vi "PMOD Example(FPGA).vi"() -> ()   [LabVIEW 2014]
uses:
  Controls/SPIExample.CurrentStateFPGA.ctl
  <userlib>/_NI SPI IP/FPGA/Controllers/Public/Transfer Settings.ctl
  vi.lib/SPIAPI/Controls/SPI Settings.ctl
  vi.lib/SPIAPI/Controls/Signal Properties.ctl
  <vilib>/rvi/Emulation/niFpgaGetClockAttributes.vi
  <vilib>/rvi/Emulation/niFpgaSctlEmulationGetInTimedLoop.vi
  <vilib>/rvi/Emulation/niFpgaEmulationReportErrorSimple.vi
  <vilib>/rvi/Emulation/niFpgaProcessEmulError.vi
  <vilib>/rvi/interface/RandomDataEmulation/niFpgaRandomDataHandleErrors.vi
  <vilib>/rvi/Emulation/niFpgaCriticalErrorInLSC.vi
  <vilib>/rvi/DataTransferAndStorage/Container/XNode/niFpgaContainer.xnode
  <vilib>/rvi/interface/RandomDataEmulation/nirviRandomDataFpgaReadWriteTemplate.vi
  <userlib>/_NI SPI IP/FPGA/Controllers/NI SPI IP FPGA.lvlib
panel:
  out "Raw ADC Data":u64
  out "read Iterations":i32
  in  "Data To ADC":u64=2147483648
  in  "Chip Select":u8
  in  "SPI PHY Settings":T1={"Divide Value"=20, "Transfer Length (bits)"=32, "CS Asserted Polarity"=FALSE, "Clock Polarity (CPOL)"=FALSE, "Clock Phase (CPHA)"=FALSE, "Lengthen MISO Setup"=FALSE, "Direction Change Bit"=0, "MOSI Starts as Output"=FALSE, "Tristatable MOSI"=FALSE} {"Direction Change Bit" max=64 step=1; "Transfer Length (bits)" min=1 max=64 step=1}
  in  "Chan Offset Array":sgl[](array[numeric])=[0.0, 0.0, 0.0, 0.0, 0.0, 0.0, 0.0, 0.0, 0.0, 0.0, 0.0, 0.0, 0.0, 0.0, 0.0, 0.0, 0.0, 0.0, 0.0, 0.0, 0.0, 0.0, 0.0, 0.0, 0.0, 0.0, 0.0, 0.0, 0.0, 0.0, 0.0, 0.0, 0.0, 0.0, 0.0, 0.0, 0.0, 0.0, 0.0, 0.0]
  out "SGL Data":sgl
  out "State":T2
  out "Iterations":i32
  in  "Debug":bool=TRUE
  out "Chan Count":bool
  out "oclk mult":u32
  in  "data rate (S/s)":u32=10000
  out "oclk freq":u32
  out "oclk div":u32
  in  "Chan Scale Array":sgl[](array[numeric])=[1.0, 1.0, 1.0, 0.0, 0.0, 0.0, 0.0, 0.0, 0.0, 0.0, 0.0, 0.0, 0.0, 0.0, 0.0, 0.0, 0.0, 0.0, 0.0, 0.0, 0.0, 0.0, 0.0, 0.0, 0.0, 0.0, 0.0, 0.0, 0.0, 0.0, 0.0, 0.0, 0.0, 0.0, 0.0, 0.0, 0.0, 0.0, 0.0, 0.0]
  out "FPGA Error":errorcluster
  out "Finished":bool
  in  "stop":bool
  out "Module Underflow":bool
  out "Acq Loop Ticks":u32
  out "DMA FIFO Full":bool
  out "First Read":bool
  in  "Number of Channels":i32=4
  in  "Acquisition Type":enum16{"Finite Samples", "Continuous Samples"}(ring)=enum."Continuous Samples"
  in  "Samps per Chan [Finite]":i32=5120
  # "OUTPUT"
  # "INPUT"
  # "ADC Data::Debug"
  # "Acquisition Parameters"
  # "SPI PHY Settings"
  # "Debug"
  # "Status"
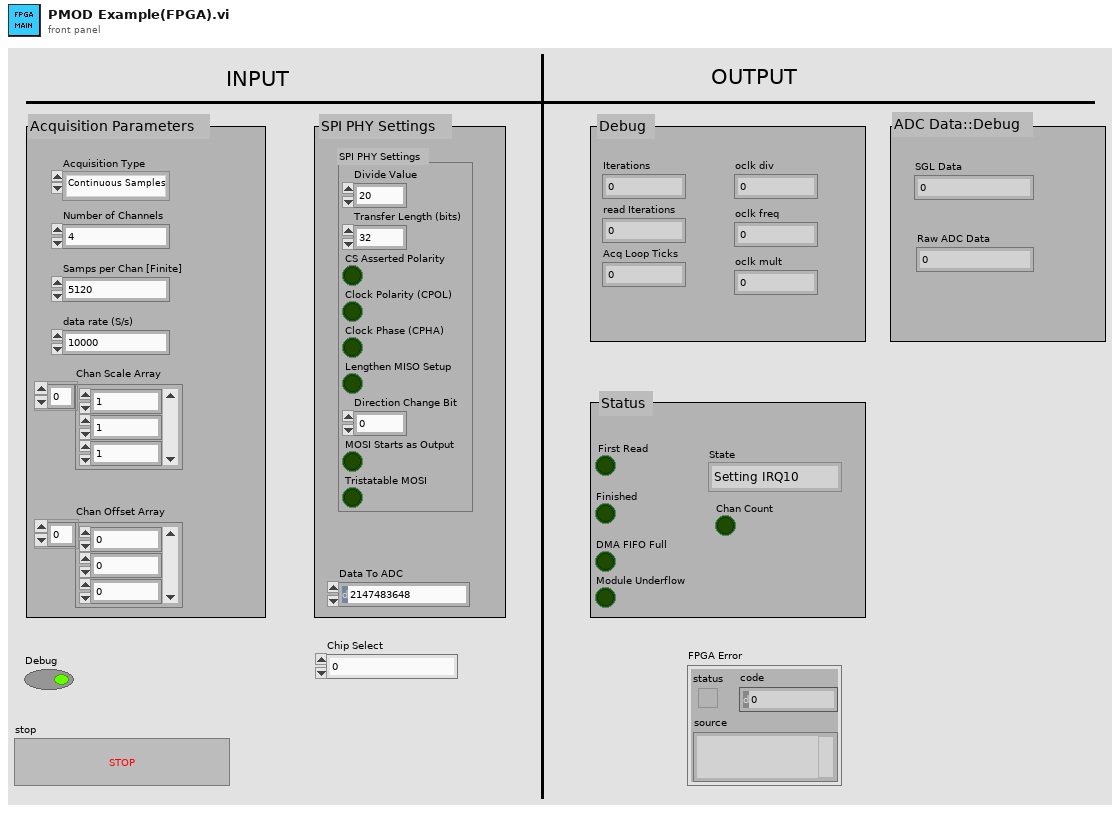
[diagram p1: front panel]
types:
  T1 = typedef "NI SPI IP FPGA.lvlib/Transfer Settings.ctl" = cluster{"Divide Value":u8, "Transfer Length (bits)":u8, "CS Asserted Polarity":bool, "Clock Polarity (CPOL)":bool, "Clock Phase (CPHA)":bool, "Lengthen MISO Setup":bool, "Direction Change Bit":u8, "MOSI Starts as Output":bool, "Tristatable MOSI":bool}
  T2 = typedef "SPIExample.CurrentStateFPGA.ctl" = enum16{"Setting IRQ10", "Config SPI", "Setting IRQ11", "Init Var", "IO Engine Running"}
  T3 = typedef "SPI Settings.ctl" = cluster{"SCLK":T4, "Signal Settings":cluster{"MISO":refnum<k21>, "Signal_Enable":refnum<k21>, "Output?":bool}, "MOSI":T4, "CS0":T4, "CS1":T4, "CS2":T4, "CS3":T4, "CS4":T4, "CS5":T4}
  T4 = typedef "Signal Properties.ctl" = cluster{"Signal":refnum<k21>, "Signal_Enable":refnum<k21>, "Output?":bool}
  T5 = typedef "All SPI Settings.ctl" = cluster{"SPI Signal Settings":T3, "SPI Internal Signals":T6, "SPI PHY Settings":T1, "SPI Engine Source":refnum<k21>}
  T6 = typedef "Internal Data (SPI API).ctl" = cluster{"DLU To SPI Engine Data FIFO":refnum<k21>, "SPI Engine to DLU Data FIFO":refnum<k21>, "Data to SPI Engine (Cache) Register":refnum<k21>, "SPI PHY Settings to SPI Engine (Cahche) Register":refnum<k21>}
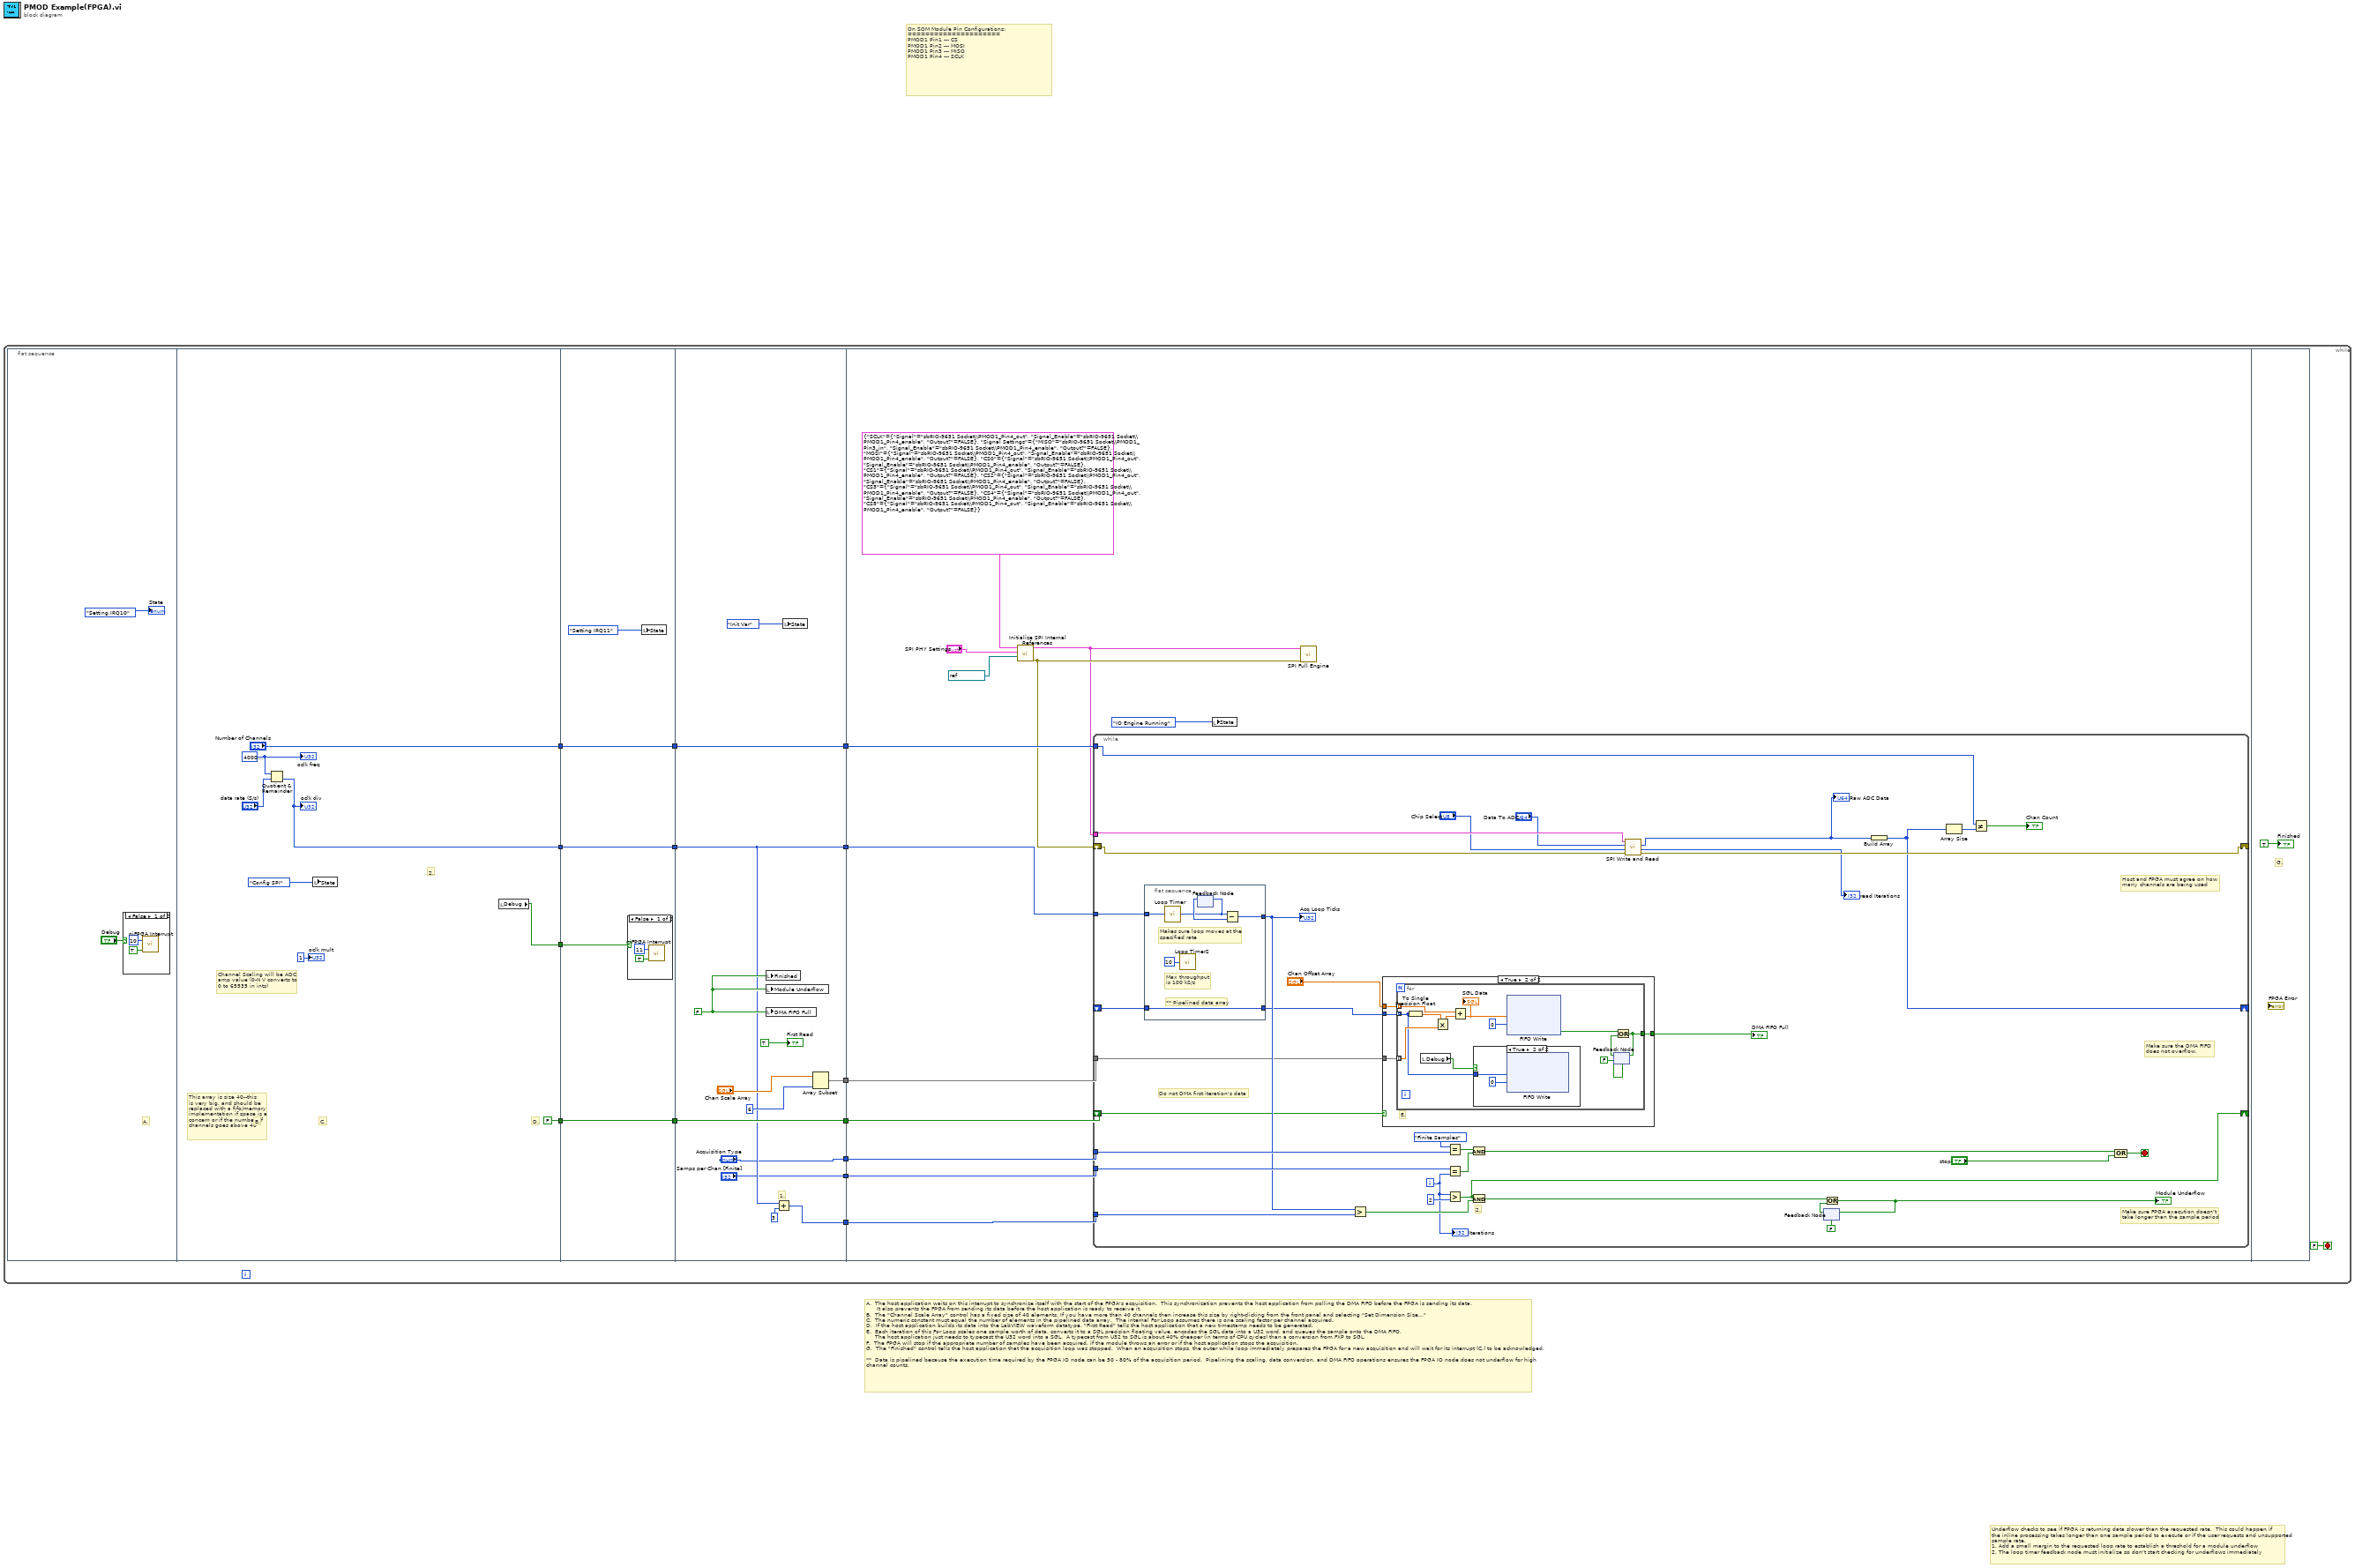
[diagram p0: block diagram]
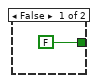
[diagram p4: hidden frame]
diagram:
  # "On SOM Module Pin Configurations:\n=====================\nPMOD1 Pin1 --- CS\nPMOD1 Pin2 --- MOSI\nPMOD1 Pin3 --- MISO\nPMOD1 Pin4 --- SCLK"
  # "Underflow checks to see if FPGA is returning data slower than the requested rate.  This could happen if\nthe inline processing takes longer than one sample period to execute or if the user requests and unsupported\nsample rate.\n1. Add a small margin to the requested loop rate to establish a threshold for a module underflow \n2. The loop timer feedback node must initialize so don't start checking for underflows immediately"
  # "A.  The host application waits on this interrupt to synchronize itself with the start of the FPGA's acquisition.  This synchronization prevents the host application from polling the DMA FIFO before the FPGA is sending its data.\n      It also prevents the FPGA from sending its data before the host application is ready to receive it.\nB.  The \"Channel Scale Array\" control has a fixed size of 40 elements. If you have more than 40 channels then increase this size by right-clicking from the front panel and selecting \"Set Dimension Size...\"\nC.  The numeric constant must equal the number of elements in the pipelined data array.  The internal For Loop assumes there is one scaling factor per channel acquired.\nD.  If the host application builds its data into the LabVIEW waveform datatype, \"First Read\" tells the host application that a new timestamp needs to be generated.\nE.  Each iteration of this For Loop scales one sample worth of data, converts it to a SGL precision floating value, encodes the SGL data into a U32 word, and queues the sample onto the DMA FIFO.  \n     The host application just needs to typecast the U32 word into a SGL.  A typecast from U32 to SGL is about 40% cheaper (in terms of CPU cycles) than a conversion from FXP to SGL.\nF.  The FPGA will stop if the appropriate number of samples have been acquired, if the module throws an error or if the host application stops the acquisition.  \nG.  The \"Finished\" control tells the host application that the acquisition loop was stopped.  When an acquisition stops, the outer while loop immediately prepares the FPGA for a new acquisition and will wait for its interrupt (C.) to be acknowledged. \n\n**  Data is pipelined because the execution time required by the FPGA IO node can be 50 - 80% of the acquisition period.  Pipelining the scaling, data conversion, and DMA FIFO operations ensures the FPGA IO node does not underflow for high\nchannel counts."
  n1 = while {
    stop <- FALSE stop-if-true
    n2 = flat-sequence {
      tunnel: ["Number of Channels"] -> w14
      tunnel: [FALSE] -> w13
      tunnel: [w23] -> w12
      tunnel: [w21] -> w1
      tunnel: w14 -> [w32]
      tunnel: [w32] -> w11
      tunnel: w13 -> [w31]
      tunnel: [w31] -> w5
      tunnel: w12 -> [w30]
      tunnel: [w30] -> w3
      tunnel: w1 -> [w29]
      tunnel: w11 -> [w47]
      tunnel: [w47] -> w10
      tunnel: [w43] -> w9
      tunnel: ["Acquisition Type"] -> w8
      tunnel: ["Samps per Chan [Finite]"] -> w7
      tunnel: [w39] -> w6
      tunnel: w5 -> [w46]
      tunnel: [w46] -> w4
      tunnel: w3 -> [w38]
      tunnel: [w38] -> w2
      tunnel: w10 -> [w60]
      tunnel: w9 -> [w58]
      tunnel: w8 -> [w57]
      tunnel: w7 -> [w56]
      tunnel: w6 -> [w55]
      tunnel: w4 -> [w54]
      tunnel: w2 -> [w59]
      frame #0 {
        # "A."
        n3 = case shown="False" "Debug" {
          frame False {
            n4 = call <vilib>:"niFPGA Interrupt.vi"("Wait Until Cleared (F)"=TRUE ("Wait Until Cleared"), "IRQ Number (0)"=u8 10 ("IRQ Number")) -> ()  [unwired: 1 in]
          }
          frame True {
          }
        }
        "State" <- SPIExample.CurrentStateFPGA."Setting IRQ10" ("State")
      }
      frame #1 {
        w24 = u32 40000000 ("oclk freq")
        # "2."
        # "This array is size 40--this\nis very big, and should be\nreplaced with a fifo/memory\nimplementation if space is a\nconcern or if the number of \nchannels goes above 40"
        # "Channel Scaling will be ADC\namp value (0-N V converts to\n0 to 65535 in ints)"
        # "D."
        # "C."
        # "B."
        n5 = Quotient & Remainder(x=w24, y="data rate (S/s)") -> (floor(x/y)=w23:u32)  [unwired: 1 out]
        "oclk div" <- w23
        n6 = local write "State"(SPIExample.CurrentStateFPGA."Config SPI" ("State")) -> ()
        n7 = local read "Debug"() -> (w21:bool)
        "oclk freq" <- w24
        "oclk mult" <- u32 1 ("oclk mult")
      }
      frame #2 {
        n8 = case shown="False" w29 {
          frame False {
            n9 = call <vilib>:"niFPGA Interrupt.vi"("Wait Until Cleared (F)"=TRUE ("Wait Until Cleared"), "IRQ Number (0)"=u8 11 ("IRQ Number")) -> ()  [unwired: 1 in]
          }
          frame True {
          }
        }
        n10 = local write "State"(SPIExample.CurrentStateFPGA."Setting IRQ11" ("State")) -> ()
      }
      frame #3 {
        w45 = FALSE ("Module Underflow")
        # "1."
        n11 = local write "Finished"(w45) -> ()
        n12 = local write "Module Underflow"(w45) -> ()
        n13 = local write "DMA FIFO Full"(w45) -> ()
        n14 = Add(x=w38, y=u32 3) -> (x+y=w39:u32)
        n15 = local write "State"(SPIExample.CurrentStateFPGA."Init Var" ("State")) -> ()
        n16 = Array Subset(array="Chan Scale Array", length=6) -> (w43:sgl[])  [unwired: 1 in]
        "First Read" <- TRUE ("First Read")
      }
      frame #4 {
        n17 = call "Initialize SPI Internal References.vi"("SPI Engine Source"=refnum<k21> "120MHz" ("Source Name"), "SPI PHY Settings"="SPI PHY Settings", "SPI Signal Settings"=T3 {"SCLK"={"Signal"="sbRIO-9651 Socket\\PMOD1_Pin4_out", "Signal_Enable"="sbRIO-9651 Socket\\PMOD1_Pin4_enable", "Output?"=FALSE}, "Signal Settings"={"MISO"="sbRIO-9651 Socket\\PMOD1_Pin3_in", "Signal_Enable"="sbRIO-9651 Socket\\PMOD1_Pin4_enable", "Output?"=FALSE}, "MOSI"={"Signal"="sbRIO-9651 Socket\\PMOD1_Pin4_out", "Signal_Enable"="sbRIO-9651 Socket\\PMOD1_Pin4_enable", "Output?"=FALSE}, "CS0"={"Signal"="sbRIO-9651 Socket\\PMOD1_Pin4_out", "Signal_Enable"="sbRIO-9651 Socket\\PMOD1_Pin4_enable", "Output?"=FALSE}, "CS1"={"Signal"="sbRIO-9651 Socket\\PMOD1_Pin4_out", "Signal_Enable"="sbRIO-9651 Socket\\PMOD1_Pin4_enable", "Output?"=FALSE}, "CS2"={"Signal"="sbRIO-9651 Socket\\PMOD1_Pin4_out", "Signal_Enable"="sbRIO-9651 Socket\\PMOD1_Pin4_enable", "Output?"=FALSE}, "CS3"={"Signal"="sbRIO-9651 Socket\\PMOD1_Pin4_out", "Signal_Enable"="sbRIO-9651 Socket\\PMOD1_Pin4_enable", "Output?"=FALSE}, "CS4"={"Signal"="sbRIO-9651 Socket\\PMOD1_Pin4_out", "Signal_Enable"="sbRIO-9651 Socket\\PMOD1_Pin4_enable", "Output?"=FALSE}, "CS5"={"Signal"="sbRIO-9651 Socket\\PMOD1_Pin4_out", "Signal_Enable"="sbRIO-9651 Socket\\PMOD1_Pin4_enable", "Output?"=FALSE}}) -> ("error out"=w52:errorcluster, "SPI Engine Reference"=w51:T5)  [unwired: 7 in]
        n18 = while {
          tunnel: w57 -> [w92]
          tunnel: w56 -> [w91]
          shift-right: [w66] -> _
          shift-left: _ -> [w85]
          tunnel: w60 -> [w70]
          tunnel: w59 -> [w90]
          tunnel: w55 -> [w87]
          tunnel: w58 -> [w75]
          shift-right: [w74] -> _
          shift-left: w54 -> [w84]
          shift-right: [w67] -> _
          shift-left: w52 -> [w68]
          tunnel: w51 -> [w63]
          i -> [w83]
          stop <- w94 stop-if-true
          # "2."
          # "Do not DMA first iteration's data"
          # "Host and FPGA must agree on how \nmany channels are being used"
          # "Make sure the DMA FIFO\ndoes not overflow."
          # "Make sure FPGA execution doesn't\ntake longer than the sample period"
          n19 = flat-sequence {
            tunnel: w90 -> [w121]
            tunnel: [w118] -> w86
            tunnel: [w117] -> w73
            tunnel: w85 -> [w117]
            frame #0 {
              # "Max throughput\nis 100 kS/s"
              # "Makes sure loop moves at the\nspecified rate"
              # "** Pipelined data array"
              n20 = call "Loop Timer"("Count(Ticks)"=w121) -> ("Tick Count(Ticks)"=w119:u32)
              n21 = call "Loop Timer2"("Count(uSec)"=u8 10 ("Count(Ticks)")) -> ()  [unwired: 1 out]
              n22 = feedback-in #1(w119) -> ()
              n23 = feedback #1() -> (w120:u32)  [unwired: 1 out]
              n24 = Subtract(x=w119, y=w120) -> (x-y=w118:u32)
            }
          }
          n25 = Greater?(x=w86, y=w87) -> (0:w89:bool)
          n26 = case shown="True" w84 {
            tunnel: [FALSE w101] -> w93
            tunnel: w73 -> [_ w100]
            tunnel: w75 -> [_ w99]
            tunnel: "Chan Offset Array" -> [_ w98]
            frame False {
            }
            frame True {
              # "E."
              n27 = for {
                tunnel: [w110] -> w101
                tunnel: w100 -> [w102] mode=indexing
                tunnel: w99 -> [w108] mode=indexing
                tunnel: w98 -> [w103] mode=indexing
                n28 = To Single Precision Float(number=w102) -> (single precision float=w106:sgl)
                n29 = local read "Debug"() -> (w105:bool)
                n30 = Multiply(x=w106, y=w108) -> (x*y=w107:sgl)
                n31 = Add(x=w103, y=w107) -> (x+y=w104:sgl)
                "SGL Data" <- w104
                n32 = case shown="True" w105 {
                  tunnel: w102 -> [_ w114]
                  frame False {
                  }
                  frame True {
                    n33 = xnode ("FIFO Write")("Element"=w114, "Timeout"=0) -> ()  [unwired: 1 in, 2 out]
                  }
                }
                n34 = xnode ("FIFO Write")("Element"=w104, "Timeout"=0) -> ("Timed Out?"=w113:bool)  [unwired: 1 in, 1 out]
                n35 = feedback #2(FALSE) -> (w111:bool)
                n36 = Or(x=w113, y=w111) -> (x .or. y?=w110:bool)
                n37 = feedback-in #2(w110) -> ()
              }
            }
          }
          "DMA FIFO Full" <- w93
          n38 = Equal?(x=enum16{"Finite Samples", "Continuous Samples"}."Finite Samples" ("y"), y=w92) -> (x = y?=w78:bool)
          n39 = Equal?(x=w91, y=w83) -> (x = y?=w77:bool)
          n40 = Greater?(x=w83, y=2) -> (0:w74:bool)
          n41 = And(x=w78, y=w77) -> (x .and. y?=w76:bool)
          n42 = And(x=w74, y=w89) -> (x .and. y?=w80:bool)
          n43 = call "SPI Write and Read.vi"("error in (no error)"=w68, "Chip Select"="Chip Select", "SPI Command"="Data To ADC", "All SPI Settings"=w63) -> ("error out"=w67:errorcluster, "Read Attempts"=→"read Iterations":i32, "SPI Return Data"=w65:u64)  [unwired: 4 in, 1 out]
          "Raw ADC Data" <- w65
          n44 = feedback #3(FALSE) -> (w82:bool)
          n45 = Or(x=w80, y=w82) -> (x .or. y?=w79:bool)
          "Module Underflow" <- w79
          n46 = feedback-in #3(w79) -> ()
          n47 = Build Array(w65) -> (w66:u64[])
          n48 = Array Size(array=w66) -> (size(s)=w72:i32)
          n49 = Not Equal?(x=w70, y=w72) -> (x != y?=→"Chan Count":bool)
          n50 = Compound Arithmetic op=OR(w76, "stop") -> (w94:bool)
          "Acq Loop Ticks" <- w86
          "Iterations" <- w83
        }
        n51 = local write "State"(SPIExample.CurrentStateFPGA."IO Engine Running" ("State")) -> ()
        n52 = call "SPI Full Engine.vi"("error in (no error)"=w52, "All SPI Settings"=w51) -> ()  [unwired: 10 in]
      }
      frame #5 {
        # "G."
        "Finished" <- TRUE ("Finished")
      }
    }
  }
